vi "Zedver_v3_ModeStringGenerator_DEFI.vi"(8 "Procesado":bool, 10 "Histograma":bool, 11 "RAW":bool) -> (2 "decimal integer string":string)   [LabVIEW 2011]
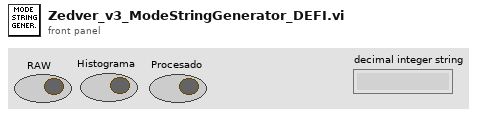
[diagram p1: front panel]
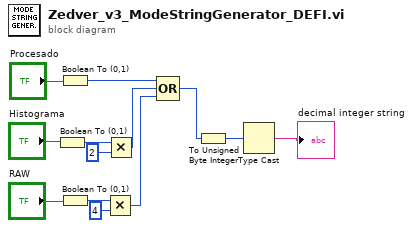
[diagram p0: block diagram]
diagram:
  n1 = Boolean To (0,1)(Boolean="Histograma") -> (0, 1=w10:i16)
  n2 = Boolean To (0,1)(Boolean="Procesado") -> (0, 1=w8:i16)
  n3 = Boolean To (0,1)(Boolean="RAW") -> (0, 1=w9:i16)
  n4 = Multiply(x=w9, y=i16 4) -> (x*y=w6:i16)
  n5 = Multiply(x=w10, y=i16 2) -> (x*y=w7:i16)
  n6 = Compound Arithmetic op=OR(w8, w7, w6) -> (w3:i16)
  n7 = To Unsigned Byte Integer(number=w3) -> (unsigned 8bit integer=w2:u8)
  n8 = Type Cast(x=w2) -> (*(type *) &x=→"decimal integer string":string)  [unwired: 1 in]
